vi "Clear Arbitrary Waveform.vi"(7 "Delete Arbitrary Waveform From Memory (False)":bool, 8 "error in (no error)":errorcluster, 10 "Arbitrary Waveform Name":string, 11 "VISA resource name":refnum<visa-resource-name>) -> (0 "error out":errorcluster, 3 "VISA resource name out":refnum<visa-resource-name>)   [LabVIEW 2015, in "Fluke 28x Series.lvlib"]
doc: "Removes a previously created arbitrary waveform from the function generator's memory. The Configure Standard Waveform VI must be called before this to change the waveform that the channel is currently displaying. Otherwise there will most likely be a \"Cannot delete arb while it is selected for any output \" error.\n\n<b>Note</b>: If <b>Delete Arbitrary Waveform from Memory</b> is False, then the waveform will only be deleted from the channel memory. If <b>Delete Arbitrary Waveform from Memory</b> is True then the waveform will be wiped from backup memory as well."
uses:
  <instrlib>/Fluke 28x Series/Fluke 28x Series.lvlib
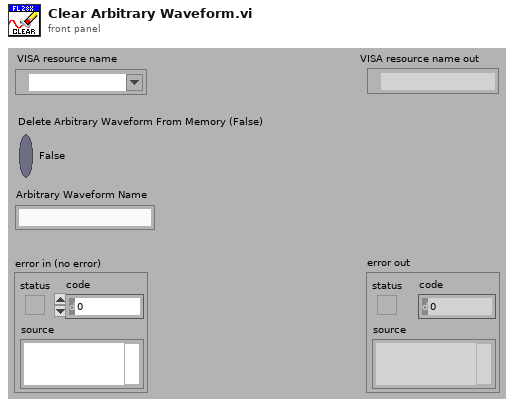
[diagram p1: front panel]
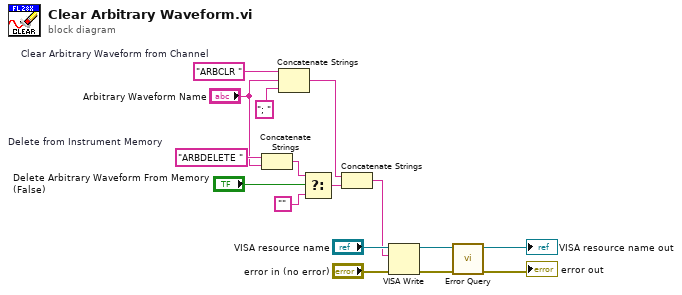
[diagram p0: block diagram]
diagram:
  w3 = "ARBDELETE "  # Delete from Instrument Memory
  w8 = "ARBCLR "  # Clear Arbitrary Waveform from Channel
  n1 = Concatenate Strings(w3, "Arbitrary Waveform Name") -> (w1:string)
  n2 = Concatenate Strings(w8, "Arbitrary Waveform Name", "; " ("string")) -> (w7:string)
  n3 = Select(t=w1, s="Delete Arbitrary Waveform From Memory (False)", f="") -> (s? t:f=w6:string)
  n4 = Concatenate Strings(w7, w6) -> (w5:string)
  n5 = VISA Write(VISA resource name="VISA resource name", write buffer=w5, error in (no error)="error in (no error)") -> (VISA resource name out=w14:refnum<visa-resource-name>, error out=w12:errorcluster)  [unwired: 1 out]
  n6 = call <instrlib>:"Error Query.vi"("error in (no error)"=w12, "VISA resource name"=w14) -> ("error out"=→"error out":errorcluster, "VISA resource name out"=→"VISA resource name out":refnum<visa-resource-name>)  [unwired: 6 in, 2 out]
